vi "Check Cell.vi"(1 "y":i32, 2 "x":i32, 3 "Grid":u8[][](array[numeric])) -> (0 "Cell":u8)   [LabVIEW 2026, in "GoL.lvlib" / "GoL.lvclass"]
uses:
  GoL.lvclass
  GoL.lvclass/GoL.ctl
panel:
  out "Window":cluster{"y":i32, "x":i32}[][](array[cluster])
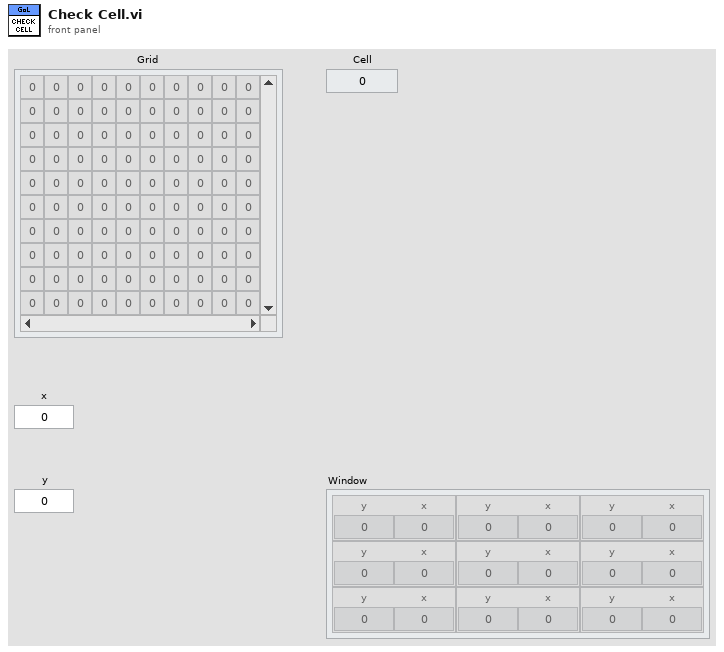
[diagram p1: front panel]
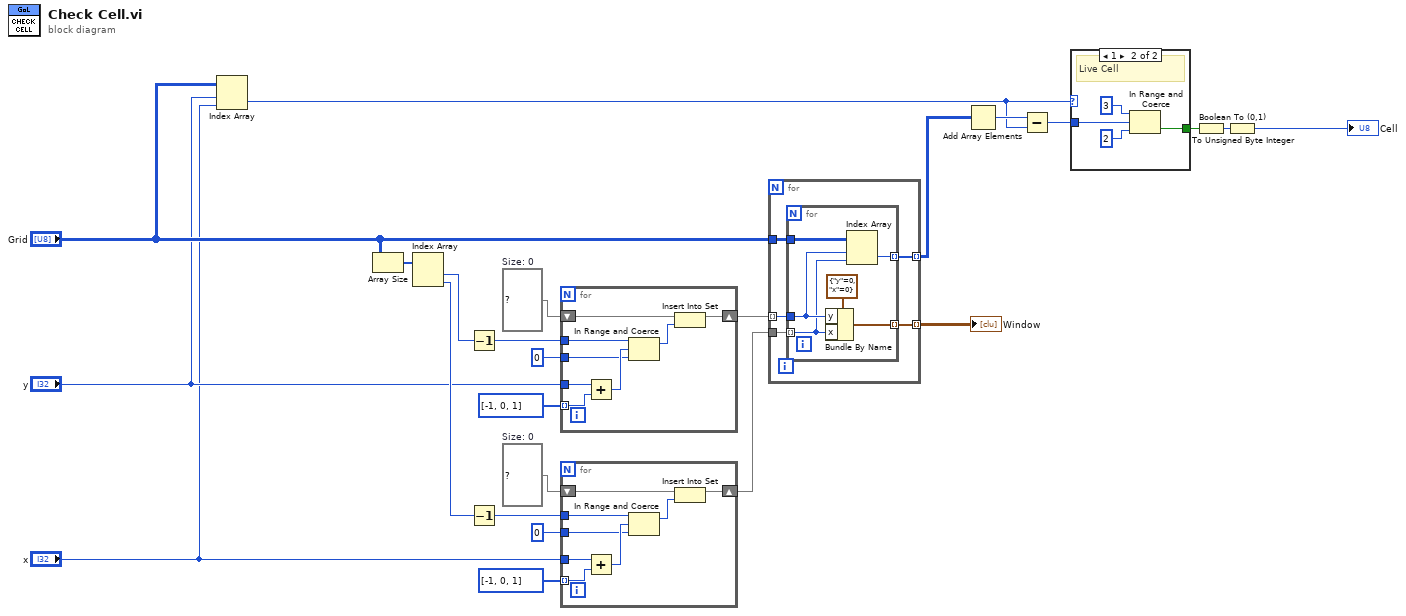
[diagram p0: block diagram]
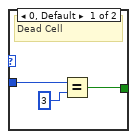
[diagram p2: hidden frame]
diagram:
  w16 = set{i32} {}  # Size: 0
  w20 = set{i32} {}  # Size: 0
  n1 = Index Array(array="Grid", index (row)="y", index (col)="x") -> (element=w2:u8)
  n2 = Array Size(array="Grid") -> (size(s)=w18:i32[])
  n3 = Index Array(array=w18) -> (element #1=w24:i32, element #2=w23:i32)  [unwired: 2 in]
  n4 = Decrement(x=w24) -> (x-1=w19:i32)
  n5 = Decrement(x=w23) -> (x-1=w17:i32)
  n6 = for {
    tunnel: i32[] [-1, 0, 1] -> [w32] mode=indexing
    tunnel: "y" -> [w31]
    tunnel: 0 ("lower limit") -> [w29]
    tunnel: w19 -> [w28]
    shift-right: [w25] -> w13
    shift-left: w20 -> [w26]
    n7 = Add(x=w31, y=w32) -> (x+y=w30:i32)
    n8 = In Range and Coerce(upper limit=w28, x=w30, lower limit=w29) -> (coerced(x)=w27:i32)  [unwired: 1 out]
    n9 = Insert Into Set(10:w27, 11:w26) -> (3:w25:set{i32})  [unwired: 1 out]
  }
  n10 = for {
    tunnel: i32[] [-1, 0, 1] -> [w40] mode=indexing
    tunnel: "x" -> [w39]
    tunnel: 0 ("lower limit") -> [w37]
    tunnel: w17 -> [w36]
    shift-right: [w33] -> w12
    shift-left: w16 -> [w34]
    n11 = Add(x=w39, y=w40) -> (x+y=w38:i32)
    n12 = In Range and Coerce(upper limit=w36, x=w38, lower limit=w37) -> (coerced(x)=w35:i32)  [unwired: 1 out]
    n13 = Insert Into Set(10:w35, 11:w34) -> (3:w33:set{i32})  [unwired: 1 out]
  }
  n14 = for {
    tunnel: w13 -> [w45] mode=indexing
    tunnel: w12 -> [w44]
    tunnel: [w43] -> w8 mode=indexing
    tunnel: [w42] -> w7 mode=indexing
    tunnel: "Grid" -> [w41]
    n15 = for {
      tunnel: w45 -> [w48]
      tunnel: w44 -> [w47] mode=indexing
      tunnel: [w50] -> w43 mode=indexing
      tunnel: w41 -> [w49]
      tunnel: [w46] -> w42 mode=indexing
      n16 = Bundle By Name(cluster=cluster{"y":i32, "x":i32} {"y"=0, "x"=0} ("Coords"), "y"=w48, "x"=w47) -> (w50:cluster{"y":i32, "x":i32})
      n17 = Index Array(array=w49, index (row)=w48, index (col)=w47) -> (element=w46:u8)
    }
  }
  "Window" <- w8
  n18 = Add Array Elements(numeric array=w7) -> (sum=w3:u8)
  n19 = Subtract(x=w3, y=w2) -> (x-y=w1:u8)
  n20 = case shown="1" w2 {
    tunnel: [w54 w56] -> w5
    tunnel: w1 -> [w53 w55]
    frame 0, Default {
      # "Dead Cell"
      n21 = Equal?(x=w53, y=u8 3) -> (x = y?=w54:bool)
    }
    frame 1 {
      # "Live Cell"
      n22 = In Range and Coerce(upper limit=u8 3, x=w55, lower limit=u8 2) -> (In Range?=w56:bool)  [unwired: 1 out]
    }
  }
  n23 = Boolean To (0,1)(Boolean=w5) -> (0, 1=w6:i16)
  n24 = To Unsigned Byte Integer(number=w6) -> (unsigned 8bit integer=→"Cell":u8)
